vi "Write ColumnIndex.vi"(8 "error in (no error)":errorcluster, 10 "ColumnIndex":i32, 11 "DataError in":refnum<class "DataError.lvclass">) -> (0 "error out":errorcluster, 3 "DataError out":refnum<class "DataError.lvclass">)   [LabVIEW 2013, in "DataGrid.lvlib" / "DataError.lvclass"]
uses:
  DataError.lvclass
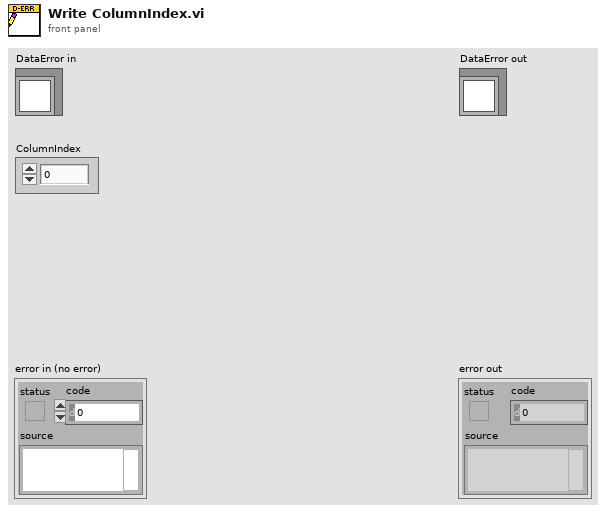
[diagram p1: front panel]
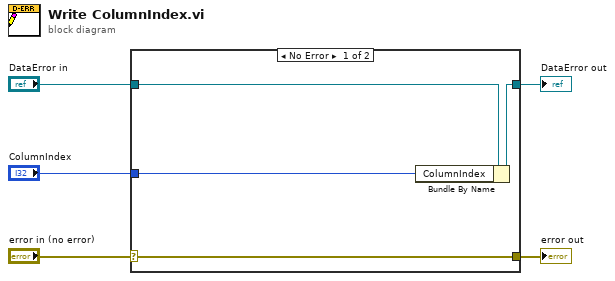
[diagram p0: block diagram]
diagram:
  n1 = case shown="No Error" "error in (no error)" {
    selector: "error in (no error)" -> [w9 w10]
    tunnel: [w9 w10] -> w4
    tunnel: [w7 w11] -> w2
    tunnel: "DataError in" -> [w8 w11]
    tunnel: "ColumnIndex" -> [w6 _]
    frame No Error {
      n2 = Bundle By Name(cluster=w8, "ColumnIndex"=w6) -> (w7:refnum<class "DataError.lvclass">)
    }
    frame Error {
    }
  }
  "error out" <- w4
  "DataError out" <- w2
